vi "Relaxation_Strength 2024.vi"(2 "Cp0 humid air / R":dbl=3.5066732874473505, 3 "C vib O2":dbl=0.23522061867822527, 4 "C vib N2":dbl=0.011869230445320268, 5 "xw molar fraction water vapor":dbl=0.01309 format="%.6g", 6 "N2 molar fraction Dry":dbl=0.780661912560544, 7 "O2 molar fraction Dry":dbl=0.20942822447048373) -> (0 "Rel strength N2":dbl=0.00012703722717918718 format="%#_6e", 1 "Rel strength O2":dbl=0.0006753922167312215 format="%#_6e")   [LabVIEW 2016]
panel:
  # "eX"
  # "eN"
  # "J mol^-1 K^-1"
  # "J mol^-1 K^-1"
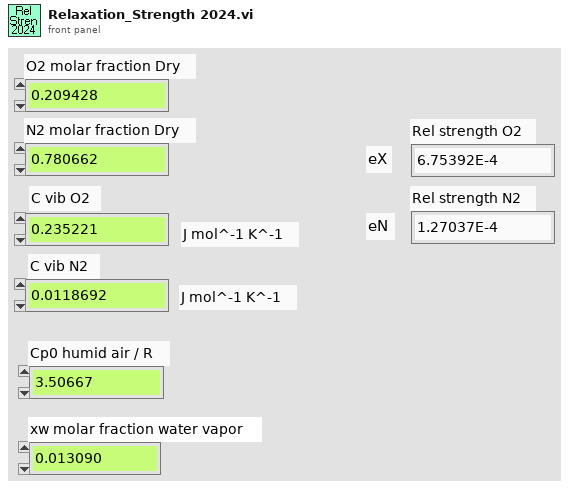
[diagram p1: front panel]
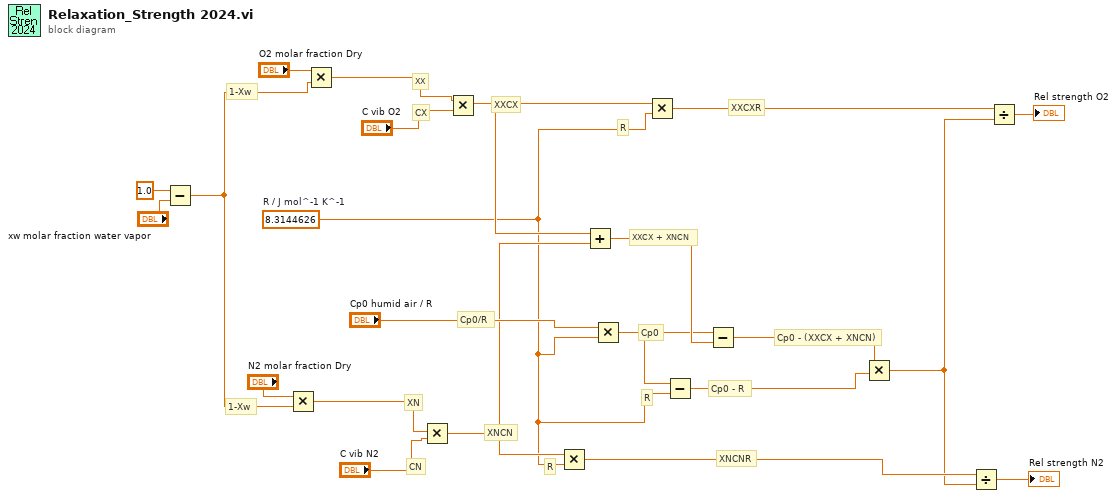
[diagram p0: block diagram]
diagram:
  w8 = 8.3144626  # R / J mol^-1 K^-1
  # "1-Xw"
  # "1-Xw"
  # "R"
  # "Cp0/R"
  # "Cp0"
  # "Cp0 - (XXCX + XNCN)"
  # "Cp0 - R"
  # "XXCX + XNCN"
  # "XNCNR"
  # "R"
  # "XNCN"
  # "XXCXR"
  # "R"
  # "XXCX"
  # "CN"
  # "CX"
  # "XN"
  # "XX"
  n1 = Subtract(x=1.0, y="xw molar fraction water vapor") -> (x-y=w1:dbl)
  n2 = Multiply(x="N2 molar fraction Dry", y=w1) -> (x*y=w3:dbl)
  n3 = Multiply(x="O2 molar fraction Dry", y=w1) -> (x*y=w4:dbl)
  n4 = Multiply(x=w3, y="C vib N2") -> (x*y=w11:dbl)
  n5 = Multiply(x=w4, y="C vib O2") -> (x*y=w19:dbl)
  n6 = Multiply(x=w11, y=w8) -> (x*y=w12:dbl)
  n7 = Add(x=w19, y=w11) -> (x+y=w17:dbl)
  n8 = Multiply(x="Cp0 humid air / R", y=w8) -> (x*y=w14:dbl)
  n9 = Multiply(x=w19, y=w8) -> (x*y=w20:dbl)
  n10 = Subtract(x=w14, y=w8) -> (x-y=w15:dbl)
  n11 = Subtract(x=w14, y=w17) -> (x-y=w16:dbl)
  n12 = Multiply(x=w16, y=w15) -> (x*y=w10:dbl)
  n13 = Divide(x=w12, y=w10) -> (x/y=→"Rel strength N2":dbl)
  n14 = Divide(x=w20, y=w10) -> (x/y=→"Rel strength O2":dbl)
